vi "start.vi"(11 "Experience ID":string) -> (0 "error out":errorcluster)   [LabVIEW 2014]
panel:
  in  "OpenFP":bool=TRUE
  # "Start"
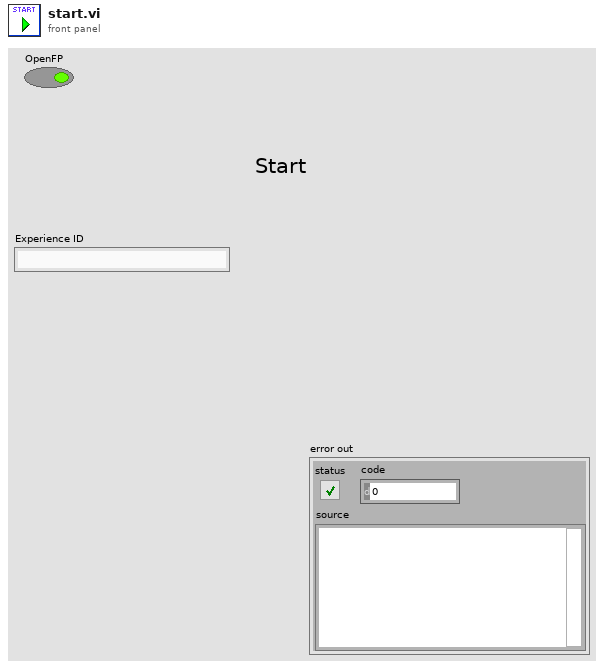
[diagram p1: front panel]
types:
  T1 = enum32{"Invalid", "Standard", "Closed", "Hidden", "Minimized", "Maximized"}
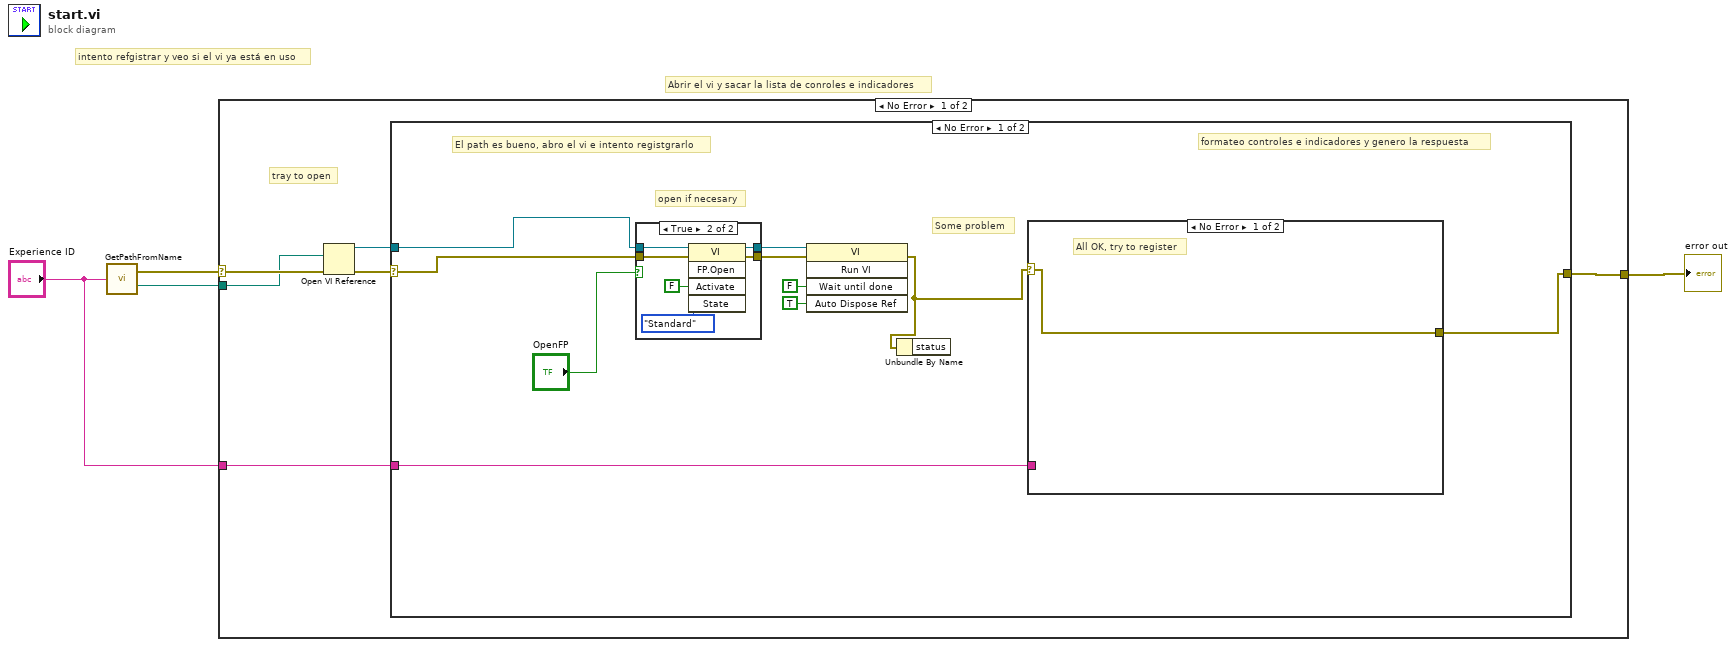
[diagram p0: block diagram]
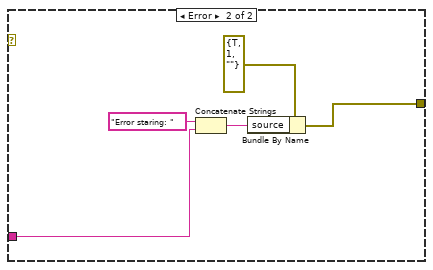
[diagram p2: hidden frame]
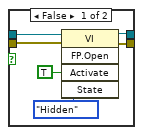
[diagram p3: hidden frame]
diagram:
  # "Abrir el vi y sacar la lista de conroles e indicadores"
  # "intento refgistrar y veo si el vi ya está en uso"
  n1 = call "GetPathFromName.vi"("Experience ID"="Experience ID") -> ("Error out"=w4:errorcluster, "VI_Path"=w3:path)
  n2 = case shown="No Error" w4 {
    selector: w4 -> [w10 w40]
    tunnel: w3 -> [w9 _]
    tunnel: "Experience ID" -> [w6 _]
    tunnel: [w5 w40] -> w1
    frame No Error {
      # "tray to open"
      n3 = Open VI Reference(vi path=w9, error in (no error)=w10) -> (vi reference=w8:refnum<vi>, error out=w7:errorcluster)  [unwired: 1 in, 3 out]
      n4 = case shown="No Error" w7 {
        selector: w7 -> [w12 w39]
        tunnel: w8 -> [w13 _]
        tunnel: w6 -> [w19 _]
        tunnel: [w18 w39] -> w5
        frame No Error {
          # "Some problem"
          # "open if necesary"
          # "formateo controles e indicadores y genero la respuesta"
          # "El path es bueno, abro el vi e intento registgrarlo"
          n5 = case shown="True" "OpenFP" {
            tunnel: w13 -> [w29 w38]
            tunnel: w12 -> [w30 w37]
            tunnel: [w31 w36] -> w16
            tunnel: [w32 w35] -> w17
            frame False {
              n6 = invoke class="VI" method="FP.Open"(reference=w29, error in=w30, "Activate"=TRUE ("Activate?"), "State"=T1."Hidden") -> (reference out=w32:refnum<vi>, error out=w31:errorcluster)  [unwired: 1 in, 3 out]
            }
            frame True {
              n7 = invoke class="VI" method="FP.Open"(reference=w38, error in=w37, "Activate"=FALSE ("Activate?"), "State"=T1."Standard") -> (reference out=w35:refnum<vi>, error out=w36:errorcluster)  [unwired: 1 in, 3 out]
            }
          }
          n8 = invoke class="VI" method="Run VI"(reference=w17, error in=w16, "Wait until done"=FALSE ("Wait Until Done"), "Auto Dispose Ref"=TRUE ("Auto Dispose Reference")) -> (error out=w11:errorcluster)  [unwired: 1 in, 4 out]
          n9 = Unbundle By Name(w11) -> ()  [unwired: 1 out]
          n10 = case shown="No Error" w11 {
            selector: w11 -> [w21 _]
            tunnel: w19 -> [_ w22]
            tunnel: [w21 w26] -> w18
            frame No Error {
              # "All OK, try to register"
            }
            frame Error {
              n11 = Concatenate Strings("Error staring: " ("string"), w22) -> (w24:string)
              n12 = Bundle By Name(cluster=errorcluster {"status"=TRUE, "code"=1, "source"=""} ("Error"), "source"=w24) -> (w26:errorcluster)
            }
          }
        }
        frame Error {
        }
      }
    }
    frame Error {
    }
  }
  "error out" <- w1
